vi "Configure.vi"(8 "error in (no error)":errorcluster, 9 "Send Pressure?":bool, 10 "NI_ChannelName":string) -> (0 "error out":errorcluster, 3 "BPG out":refnum<class "BPG.lvclass">)   [LabVIEW 2021, in "BPG.lvclass"]
uses:
  BPG.lvclass
  BPG.lvclass/BPG.ctl
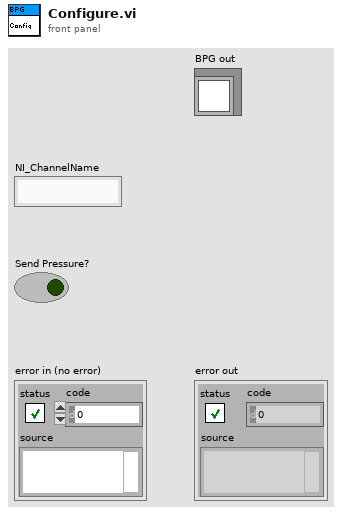
[diagram p1: front panel]
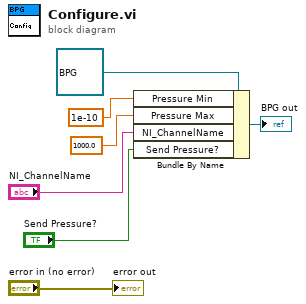
[diagram p0: block diagram]
diagram:
  n1 = Bundle By Name(cluster=refnum<class "BPG.lvclass"> refnum ("BPG.lvlib:BPG.lvclass"), "Pressure Min"=1e-10, "Pressure Max"=1000.0, "NI_ChannelName"="NI_ChannelName", "Send Pressure?"="Send Pressure?") -> (→"BPG out":refnum<class "BPG.lvclass">)
  "error out" <- "error in (no error)"
